vi "Prepare.vi"(8 "error in (no error)":errorcluster) -> (0 "error out":errorcluster, 2 "Owner":refnum<vi>, 3 "vi refnum":refnum<vi>)   [LabVIEW 2018, in "JSON to LVConstant Test.lvlib"]
uses:
  JSON to LVConstant Test.lvlib
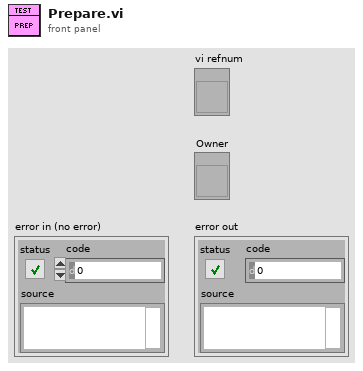
[diagram p1: front panel]
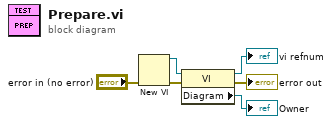
[diagram p0: block diagram]
diagram:
  n1 = New VI(8:"error in (no error)") -> (0:w1:errorcluster, 3:w3:refnum<vi>)  [unwired: 6 in]
  n2 = property on="Property Node" class="VI"(reference=w3, error in=w1) -> (reference out=→"vi refnum":refnum<vi>, error out=→"error out":errorcluster, "Diagram"=→"Owner":refnum<vi>)
